vi "find flat instance.vi"(8 "error in":errorcluster, 10 "ID":string, 11 "flat hierarchy":T2) -> (0 "error out":errorcluster, 3 "instancedata":T1)   [LabVIEW 2013, in "NISE_CEF_TreeSerializer.lvlib"]
doc: "Searches a flattened instance set for the instance with a given ID."
uses:
  NISE_CEF_TreeSerializer.lvlib
  flat hierarchy.ctl
  full hierarchy.ctl
  hierarchy element.ctl
  instance data.ctl
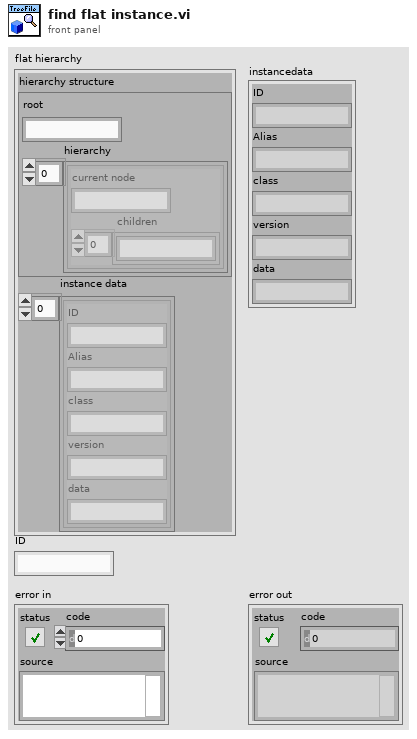
[diagram p1: front panel]
types:
  T1 = typedef "NISE_CEF_TreeSerializer.lvlib/instance data.ctl" = cluster{"ID":string, "Alias":string, "class":string, "version":string, "data":string}
  T2 = typedef "NISE_CEF_TreeSerializer.lvlib/flat hierarchy.ctl" = cluster{"hierarchy structure":T3, "instance data":T1[]}
  T3 = typedef "NISE_CEF_TreeSerializer.lvlib/full hierarchy.ctl" = cluster{"root":string, "hierarchy":T4[]}
  T4 = typedef "NISE_CEF_TreeSerializer.lvlib/hierarchy element.ctl" = cluster{"current node":string, "children":string[]}
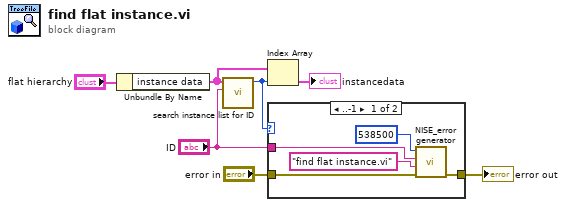
[diagram p0: block diagram]
diagram:
  n1 = Unbundle By Name("flat hierarchy") -> ("instance data"=w6:T1[])
  n2 = call "search instance list for ID.vi"("UID"="ID", "instance data"=w6) -> ("index"=w4:i32)  [unwired: 9 in]
  n3 = Index Array(array=w6, index=w4) -> (element=→"instancedata":T1)
  n4 = case shown="..-1" w4 {
    tunnel: [w11 w13] -> w3
    tunnel: "error in" -> [w12 w13]
    tunnel: "ID" -> [w9 _]
    frame ..-1 {
      n5 = call "NISE_error generator.vi"("error in"=w12, "source"="find flat instance.vi", "append error message"=w9, "error code (0)"=538500) -> ("error out"=w11:errorcluster)  [unwired: 5 in]
    }
    frame 0.. {
    }
  }
  "error out" <- w3
